vi "MAIN_HGB2_rev04.vi"() -> ()   [LabVIEW 2016]
uses:
  Producer_Case_Structure.ctl
  Consumer Control.ctl
  <vilib>/Utility/error.llb/DialogType.ctl
  <vilib>/DAQmx/write.llb/DAQmx Write (Analog 1D DBL NChan 1Samp).vi
  <vilib>/DAQmx/miscellaneous.llb/DAQmx Fill In Error Info.vi
  <vilib>/express/express analysis/Spectral/Block/exnSpectralBlock spectral measurements RMS poly.vi
  <vilib>/express/express analysis/Spectral/Block/exnSpectralBlock spectral measurements RMS array WFM.vi
  <vilib>/express/express analysis/Spectral/XNode/ExpressSpectralMeasurementsBlockNode.xnode
panel:
  in  "Dummy Variable 2":dbl=100.0
  in  "Evaluate\nShutdown\nCriteria":bool
  out "TDMS":i32=28826
  out "Acc":i32
  in  "Numeric":i32
  out "Producer":i32=163974
  out "Control":i32=5963
  in  "Speed Setpoint":dbl
  in  "Operator Notes":string
  in  "Dummy Variable":dbl
  in  "Record Data":bool
  in  "Sample Rate [S/s]":dbl=10.0
  in  "file path":path=path "C:/LabVIEW/TDMS Data/raw/090921-LifeTest1.tdms"
  in  "Stop":bool
  in  "Tab Control":T1(tab)=enum."Pressure & Temperature"
  out "System Temperatures":waveform(dbl)[](graph)=[{"t0"=timestamp(3713989500.4597507 s since 1904-01-01), "dt"=0.1, "Y"=[59.13780420730835, 59.13780420730835, 59.13780420730835, 59.13780420730835, 59.13780420730835], "attributes"=variant("NI_ChannelName"=variant(string "T_dis_dwnstrm"), "NI_UnitDescription"=variant(string "Deg C"))}, {"t0"=timestamp(3713989500.4597507 s since 1904-01-01), "dt"=0.1, "Y"=[19.89625827807839, 19.89625827807839, 19.89625827807839, 19.89625827807839, 19.89625827807839], "attributes"=variant("NI_ChannelName"=variant(string "T_liq"), "NI_UnitDescription"=variant(string "Deg C"))}, {"t0"=timestamp(3713989500.4597507 s since 1904-01-01), "dt"=0.1, "Y"=[51.99833247781037, 51.99833247781037, 51.99833247781037, 51.99833247781037, 51.99833247781037], "attributes"=variant("NI_ChannelName"=variant(string "T_gas_mix"), "NI_UnitDescription"=variant(string "Deg C"))}, {"t0"=timestamp(3713989500.4597507 s since 1904-01-01), "dt"=0.1, "Y"=[19.22760588195371, 19.22760588195371, 19.22760588195371, 19.22760588195371, 19.22760588195371], "attributes"=variant("NI_ChannelName"=variant(string "T_wf_cd_out"), "NI_UnitDescription"=variant(string "Deg C"))}, {"t0"=timestamp(3713989500.4597507 s since 1904-01-01), "dt"=0.1, "Y"=[18.627060719483154, 18.627060719483154, 18.627060719483154, 18.627060719483154, 18.627060719483154], "attributes"=variant("NI_ChannelName"=variant(string "T_cf_in"), "NI_UnitDescription"=variant(string "Deg C"))}]
  out "System Pressures":waveform(dbl)[](graph)=[{"t0"=timestamp(3713989500.4597507 s since 1904-01-01), "dt"=0.1, "Y"=[578.0486646128056, 578.0682722227018, 578.1264189279104, 578.222428603953, 578.1051210068165], "attributes"=variant("NI_ChannelName"=variant(string "P_comp_suc"))}, {"t0"=timestamp(3713989500.4597507 s since 1904-01-01), "dt"=0.1, "Y"=[583.306176195375, 583.3785215845983, 583.209828363933, 583.2270695548225, 583.3612803937087], "attributes"=variant("NI_ChannelName"=variant(string "P_comp_dis"))}, {"t0"=timestamp(3713989500.4597507 s since 1904-01-01), "dt"=0.1, "Y"=[578.9482116510878, 578.9603819034805, 578.9117008939097, 578.9999352237569, 578.9603819034805], "attributes"=variant("NI_ChannelName"=variant(string "P_comp_int"))}]
  out "Mass Flow":waveform(dbl)(graph)={"t0"=timestamp(3713989500.4597507 s since 1904-01-01), "dt"=0.1, "Y"=[-2.9024525025681674e-05, -2.9024525025681674e-05, -2.884801084886493e-05, -2.874504424572183e-05, -2.8818591819395473e-05], "attributes"=variant("NI_ChannelName"=variant(string "m_dot_wf"))}
  out "Setpoint Temperatures":waveform(dbl)[](graph)=[{"t0"=timestamp(3713989500.4597507 s since 1904-01-01), "dt"=0.1, "Y"=[31.196546478325374, 31.196546478325374, 31.196546478325374, 31.196546478325374, 31.196546478325374], "attributes"=variant("NI_ChannelName"=variant(string "T_comp_suc"), "NI_UnitDescription"=variant(string "Deg C"))}, {"t0"=timestamp(3713989500.4597507 s since 1904-01-01), "dt"=0.1, "Y"=[50.404968165402465, 50.404968165402465, 50.404968165402465, 50.404968165402465, 50.404968165402465], "attributes"=variant("NI_ChannelName"=variant(string "T_comp_out"), "NI_UnitDescription"=variant(string "Deg C"))}, {"t0"=timestamp(3713989500.4597507 s since 1904-01-01), "dt"=0.1, "Y"=[10.877218299088199, 10.876120226653185, 10.872864039787359, 10.867488088099194, 10.874056684092338], "attributes"=variant("NI_ChannelName"=variant(string "Suc_Suph"), "NI_UnitDescription"=variant(string "Deg C"))}]
  out "Power Constituents":waveform(dbl)[](graph)=[{"t0"=timestamp(3713989500.4597507 s since 1904-01-01), "dt"=0.1, "Y"=[-0.3841233029528297, -0.3841233029528297, -0.38402523952126444, -0.384466524963301, -0.3847116835422213], "attributes"=variant("NI_ChannelName"=variant(string "Voltage"))}, {"t0"=timestamp(3713989500.4597507 s since 1904-01-01), "dt"=0.1, "Y"=[-0.033083011419059005, -0.033507952955837084, -0.03358967248214029, -0.03337720171375125, -0.03327913828218598], "attributes"=variant("NI_ChannelName"=variant(string "Frequency"))}, {"t0"=timestamp(3713989499.86075 s since 1904-01-01), "dt"=0.1, "Y"=[0.07524272613227367, 0.09587410651147366, 0.12166333198547363, 0.09587410651147366, 0.07524272613227367], "attributes"=variant("NI_ChannelName"=variant(string "Torque"))}, {"t0"=timestamp(3713989499.910749 s since 1904-01-01), "dt"=0.1, "Y"=[-11.165670305490494, 3.2762959599494934, 13.591986149549484, 13.591986149549484, 1.2131579220294952], "attributes"=variant("NI_ChannelName"=variant(string "Tachometer"))}]
  out "Raw Acceleration":waveform(dbl)[](graph)
  out "Accel. Spectrum":cluster{"f0":dbl, "df":dbl, "magnitude":dbl[]}[](graph)
  in  "?":path=path "C:/Users/ASITest/Desktop/REFPROP"
  in  "Working Fluid":string="R134A.FLD"
  # "Stop VI"
  # "Air Squared Hot Gas Bypass Test Stand"
  # "Point to where REFPROP is..."
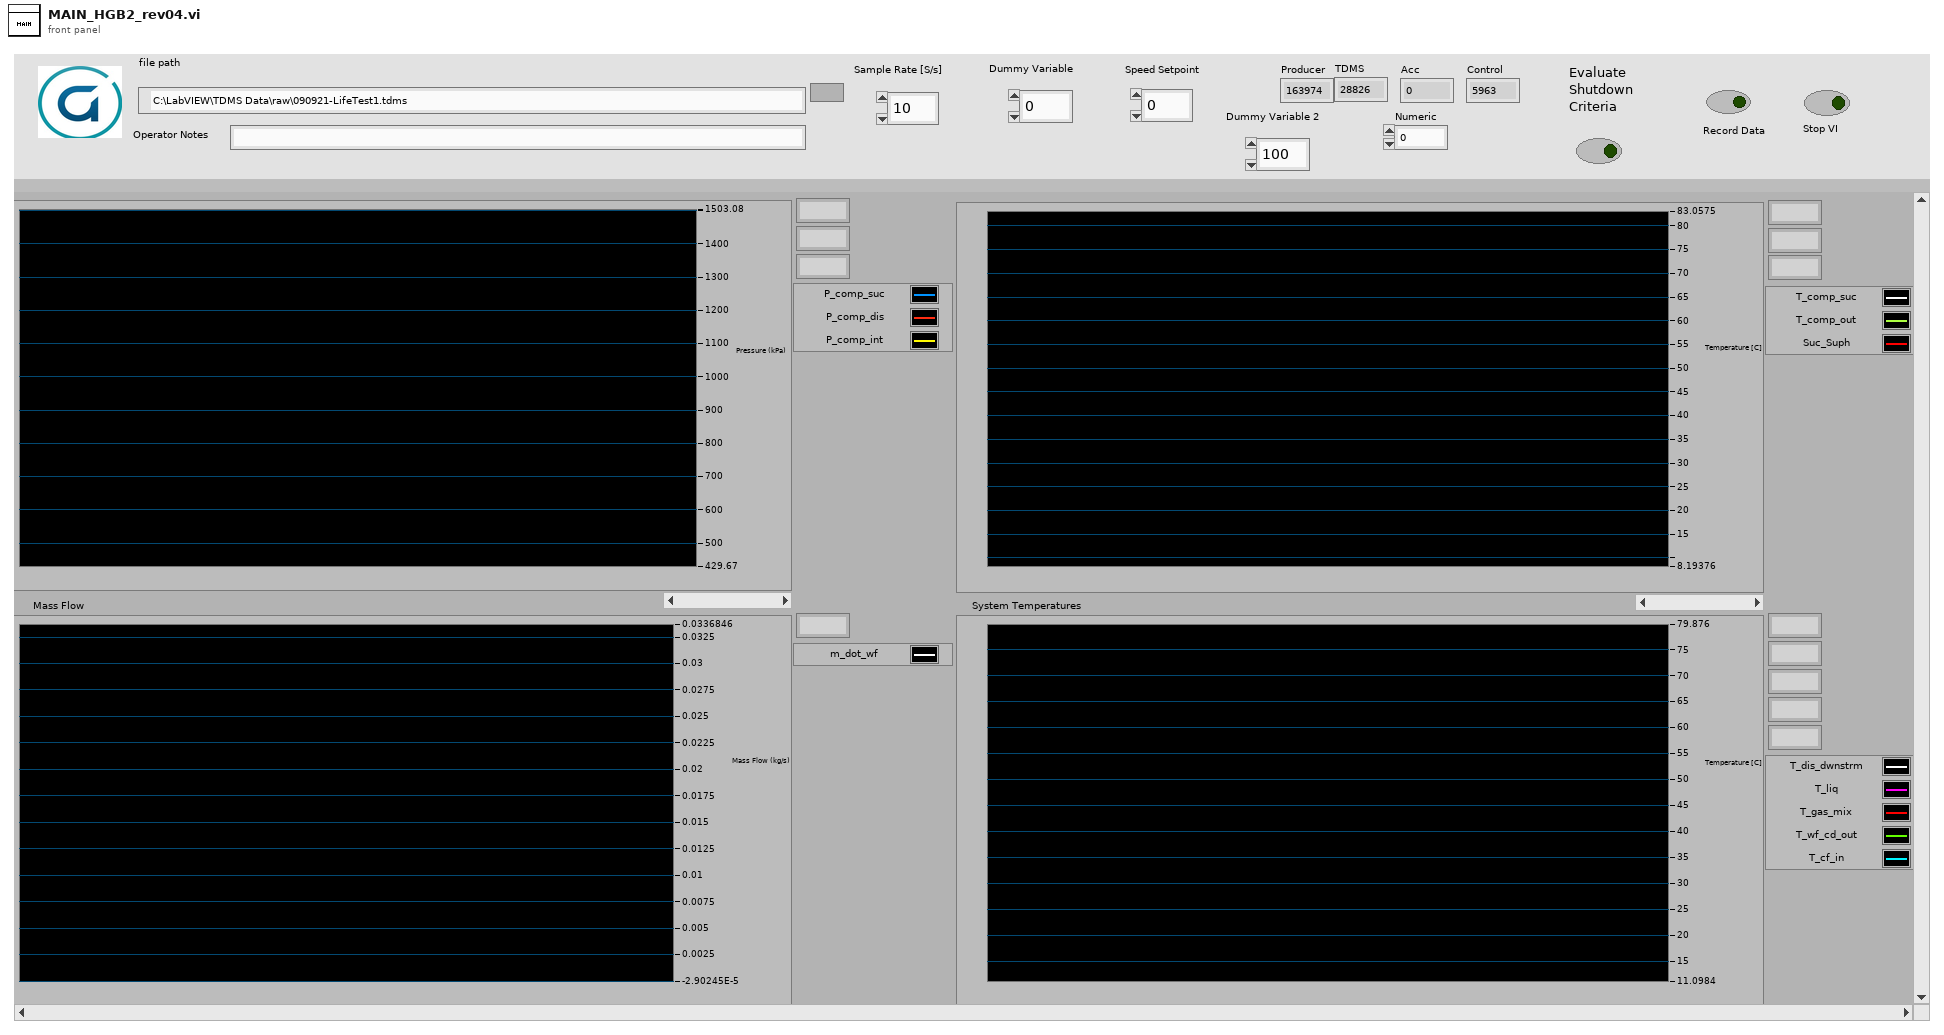
[diagram p1: front panel]
types:
  T1 = enum32{"Schematic", "Pressure & Temperature", "Power", "Acceleration", "Efficiency"}
  T2 = typedef "Consumer Control.ctl" = enum16{"System Run", "Shutdown"}
  T3 = enum16{"open", "open or create", "create or replace", "create", "open (read-only)"}
  T4 = typedef "Producer_Case_Structure.ctl" = enum16{"Initialize", "Read", "Write", "Display", "Queue", "Evaluate", "Error", "Shutdown"}
  T5 = cluster{"Data Main":waveform(dbl)[], "Accelerometer":waveform(dbl)[], "Dummy Variable":dbl, "Operator Notes":string, "Speed Setpoint":dbl, "NI 6001":waveform(dbl)[], "On/Off":dbl}
  T6 = typedef "DialogType.ctl" = u16
  T7 = cluster{"averaging mode":u16, "weighting mode":u16, "number of averages":u32}
  T8 = cluster{"dB On (F)":bool, "unwrap phase (F)":bool, "convert to degree (F)":bool}
  T9 = cluster{"All Channels":tag[], "All Labels":string[], "All Units":string[], "Slope":dbl[], "Y-Intercept":dbl[]}
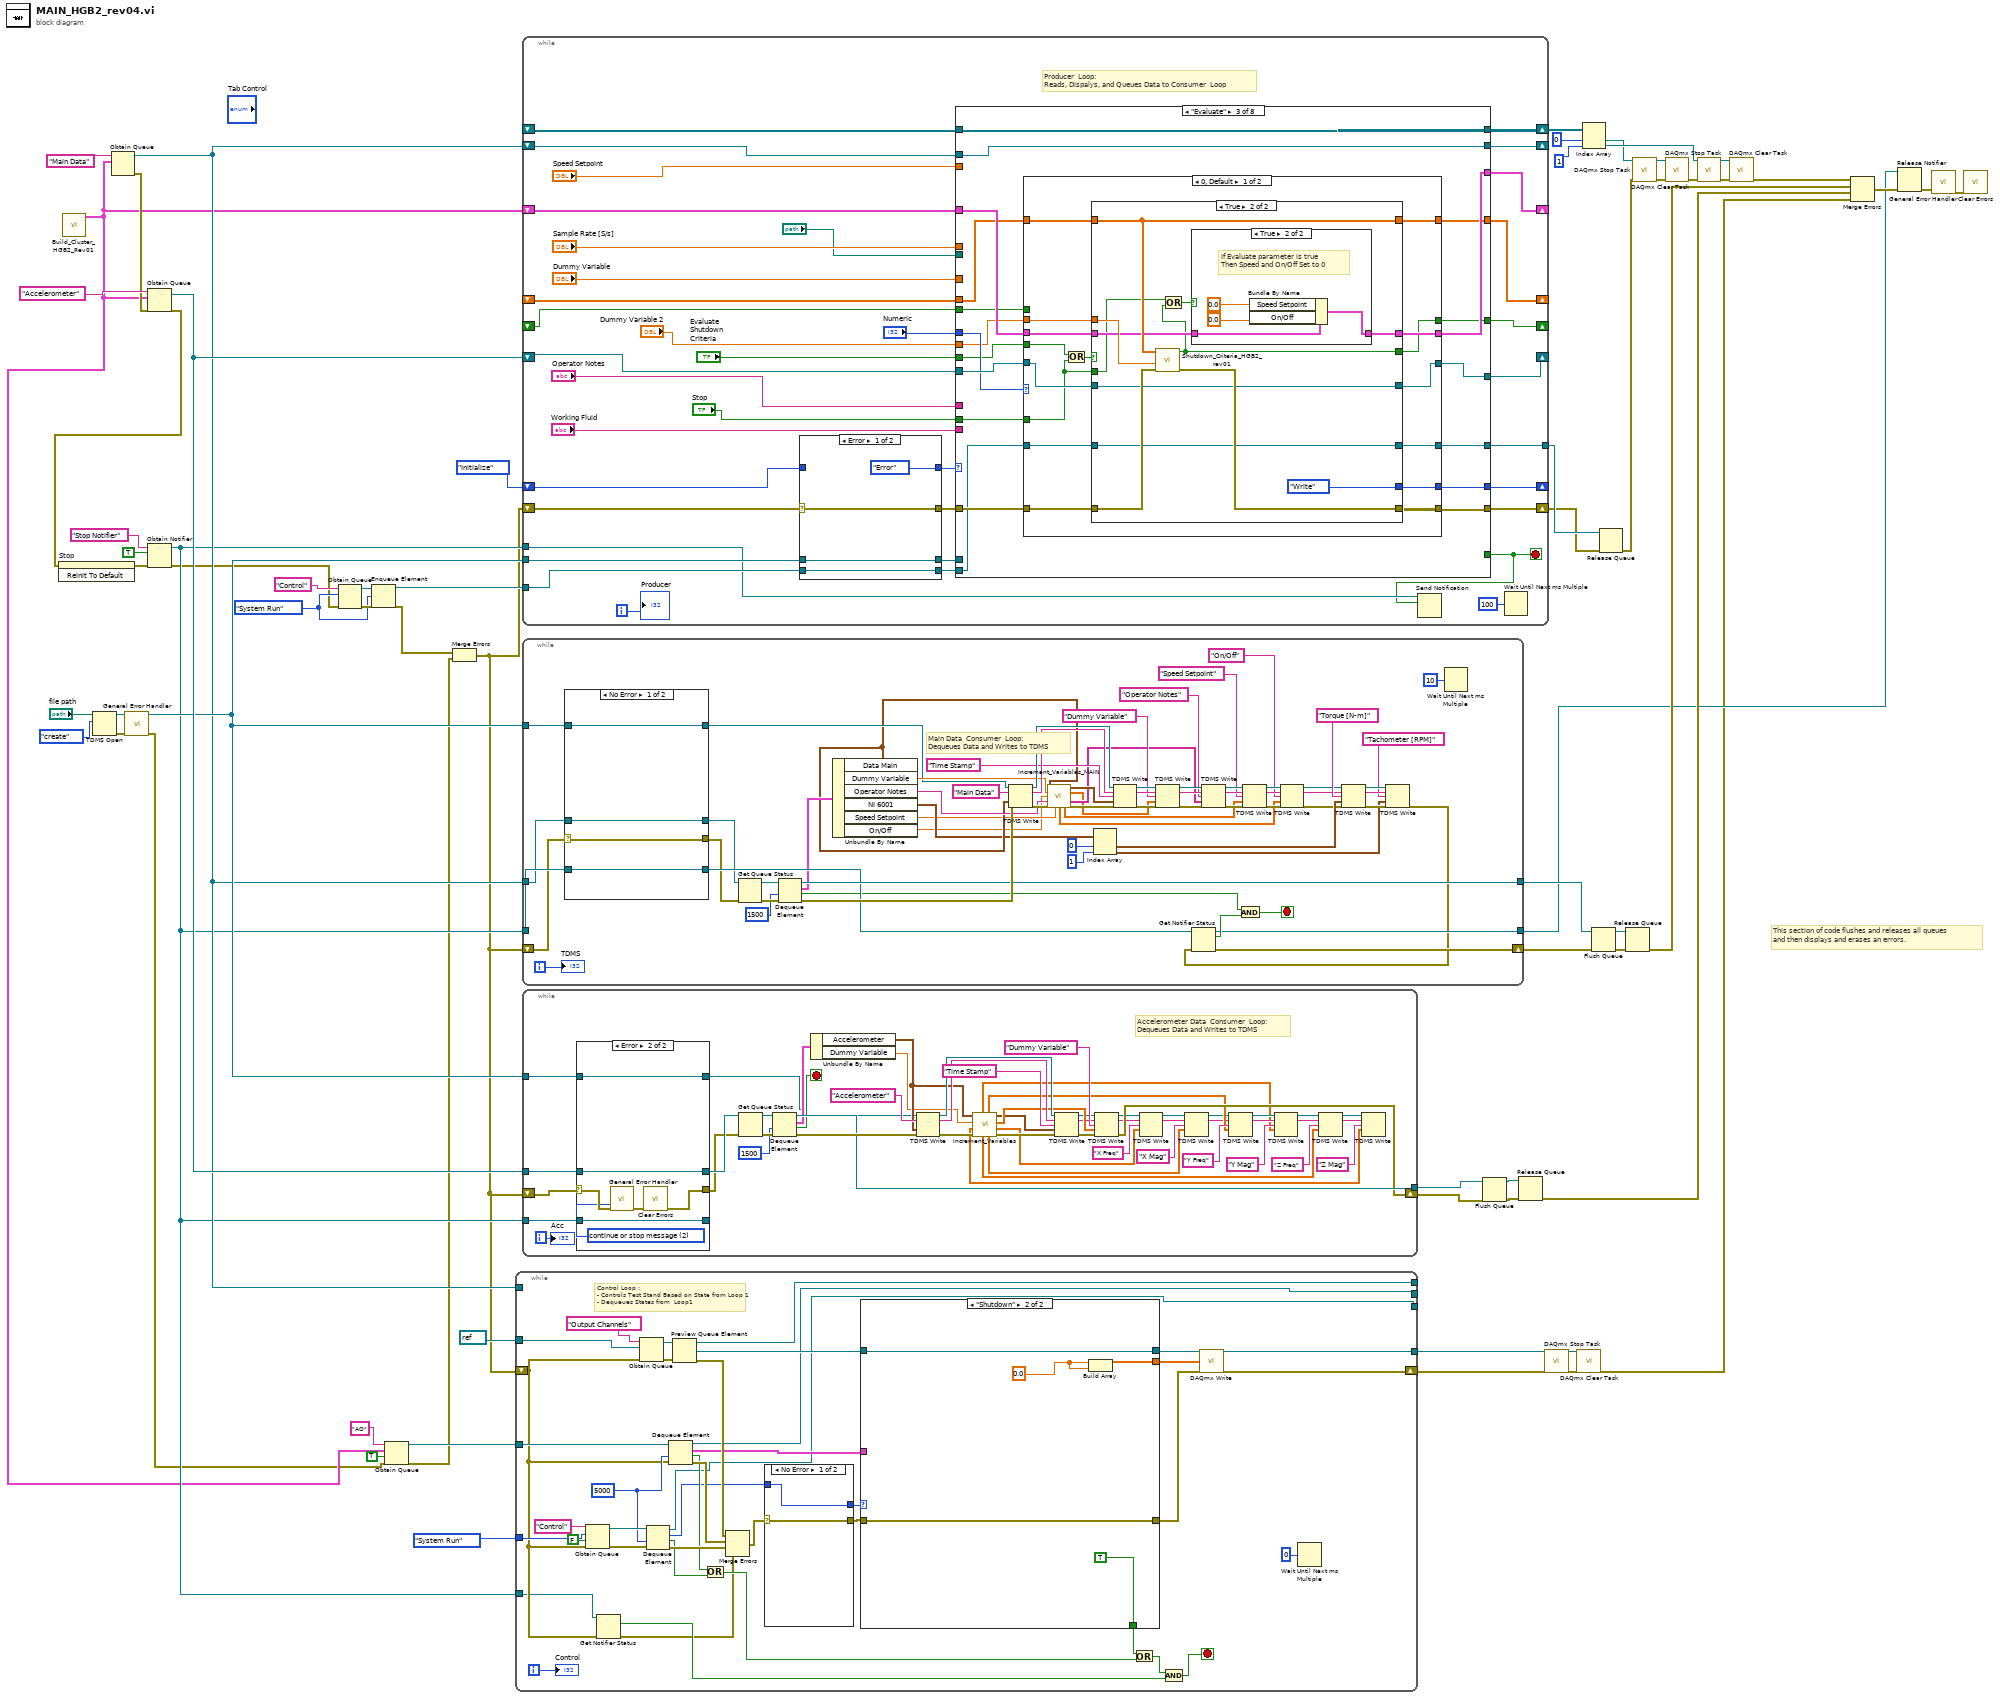
[diagram p0: block diagram]
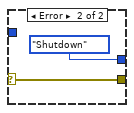
[diagram p2: hidden frame]
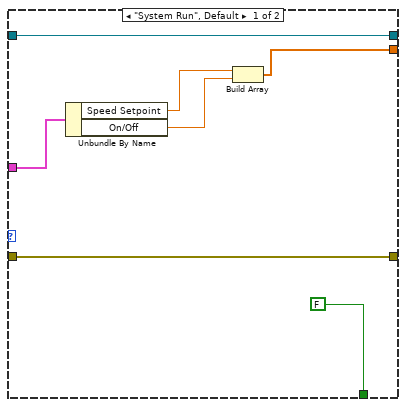
[diagram p3: hidden frame]
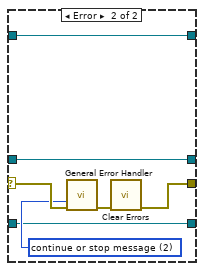
[diagram p5: hidden frame]
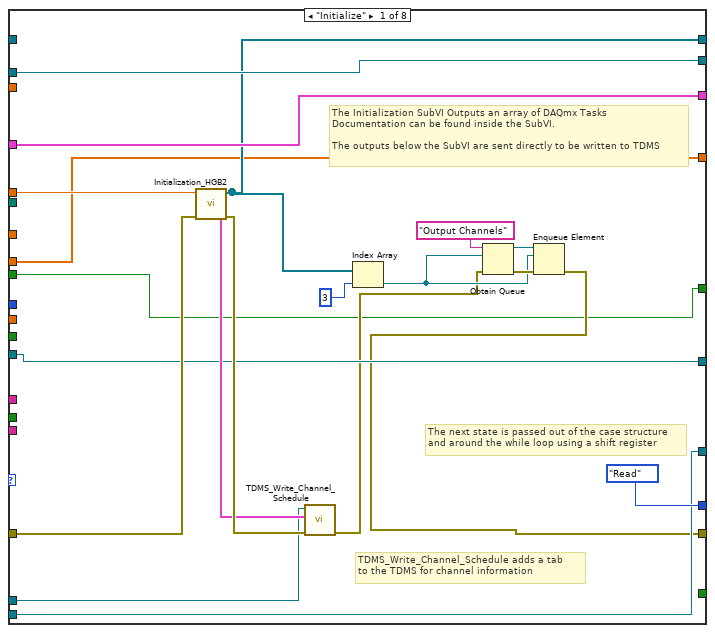
[diagram p6: hidden frame]
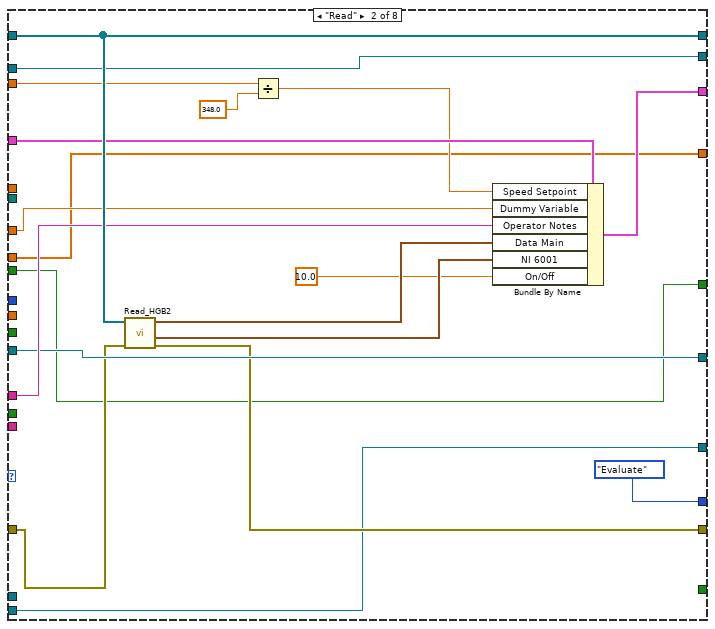
[diagram p7: hidden frame]
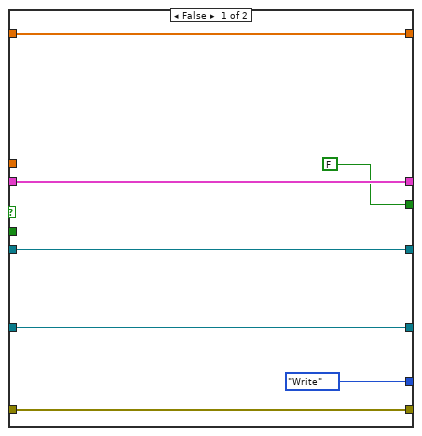
[diagram p8: hidden frame]
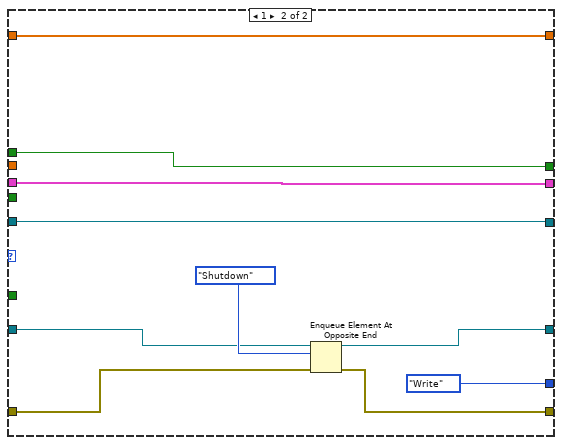
[diagram p10: hidden frame]
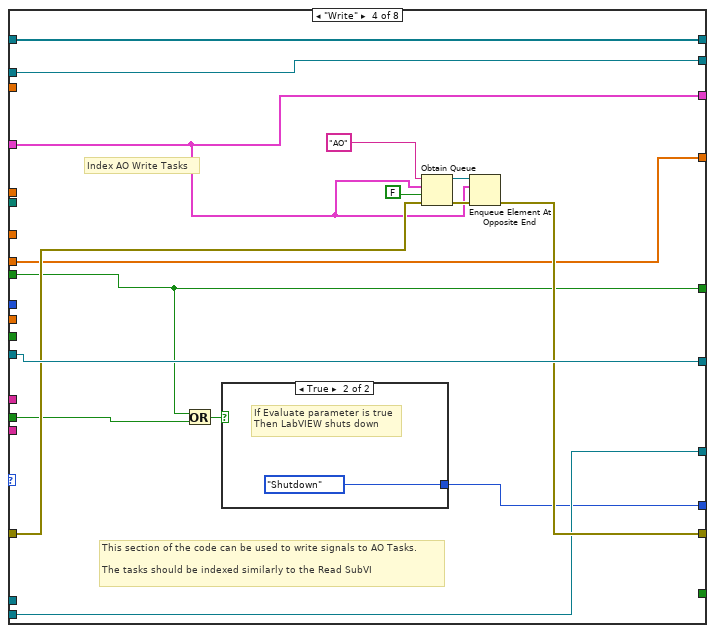
[diagram p11: hidden frame]
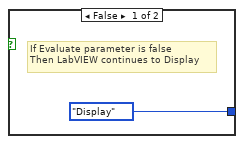
[diagram p12: hidden frame]
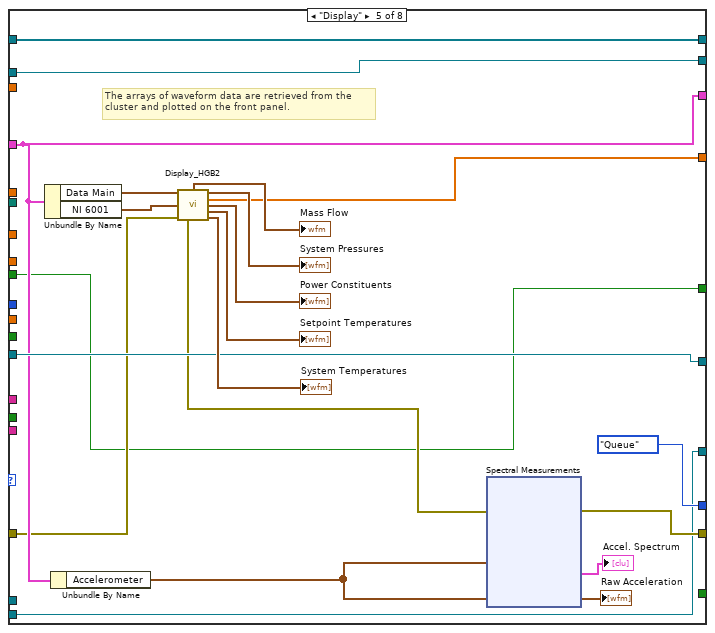
[diagram p13: hidden frame]
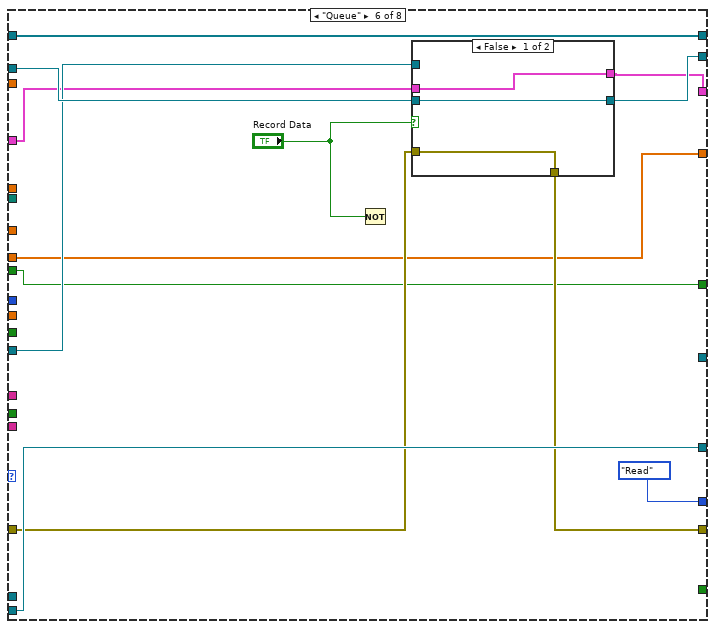
[diagram p14: hidden frame]
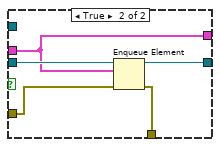
[diagram p15: hidden frame]
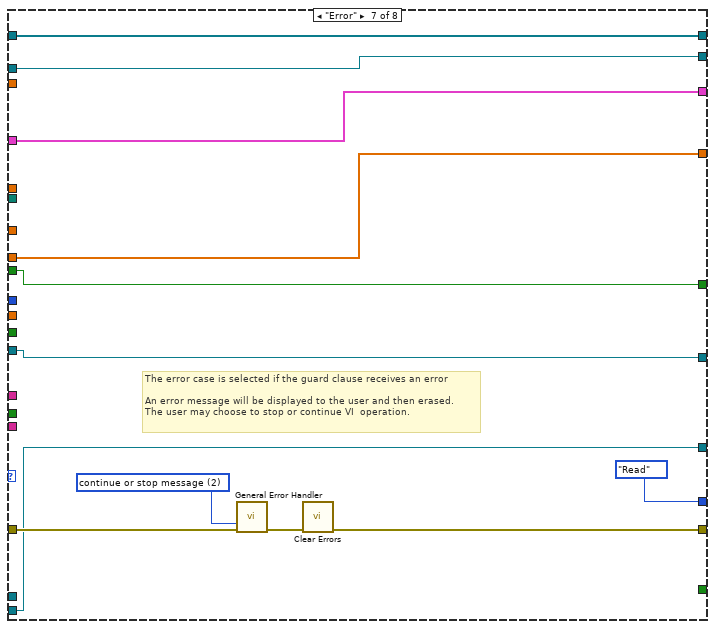
[diagram p16: hidden frame]
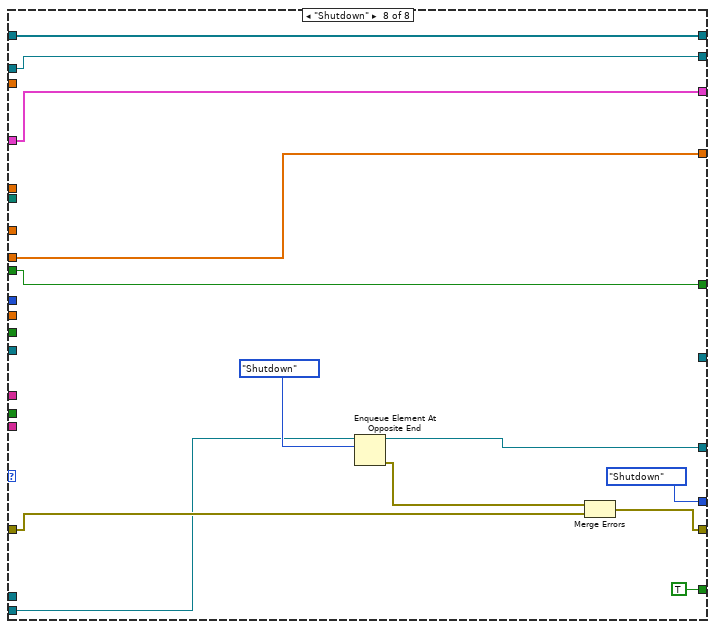
[diagram p17: hidden frame]
diagram:
  w21 = Consumer_Control."System Run"
  # "This section of code flushes and releases all queues \nand then displays and erases an errors."
  n1 = call "Build_Cluster_HGB2_Rev01.vi"() -> ("output cluster"=w13:T5)  [unwired: 11 in]
  n2 = TDMS Open(10:T3."create" ("operation (0:open)"), 11:"file path") -> (0:w54:errorcluster, 3:w37:refnum<k34>)  [unwired: 5 in]
  n3 = Obtain Queue(name (unnamed)="Main Data", element data type=w13) -> (queue out=w34:refnum<queue>, error out=w43:errorcluster)  [unwired: 3 in, 1 out]
  n4 = call <vilib>:"General Error Handler.vi"("error in (no error)"=w54) -> ("error out"=w12:errorcluster)  [unwired: 10 in, 4 out]
  n5 = Obtain Queue(name (unnamed)="Accelerometer", element data type=w13, error in (no error)=w43) -> (queue out=w42:refnum<queue>, error out=w11:errorcluster)  [unwired: 2 in, 1 out]
  n6 = invoke on="Stop" class="Bool (strict)" method="Reinit To Default"(error in=w11) -> (error out=w59:errorcluster)  [unwired: 2 in, 2 out]
  n7 = Obtain Notifier(name (unnamed)="Stop Notifier", notification data type=TRUE, error in (no error)=w59) -> (notifier out=w30:refnum<notifier>, error out=w10:errorcluster)  [unwired: 1 in, 1 out]
  n8 = Obtain Queue(name (unnamed)="Control", element data type=w21, error in (no error)=w10) -> (queue out=w23:refnum<queue>, error out=w22:errorcluster)  [unwired: 2 in, 1 out]
  n9 = Enqueue Element(queue=w23, element=w21, error in (no error)=w22) -> (queue out=w20:refnum<queue>, error out=w8:errorcluster)  [unwired: 1 in, 1 out]
  n10 = Obtain Queue(name (unnamed)="AO", element data type=w13, create if not found? (T)=TRUE, error in (no error)=w12) -> (queue out=w14:refnum<queue>, error out=w7:errorcluster)  [unwired: 1 in, 1 out]
  n11 = Merge Errors(w8, w7) -> (w9:errorcluster)
  n12 = while {
    tunnel: [w102] -> w4
    shift-right: [w89] -> w3
    shift-left: w9 -> [w70]
    tunnel: refnum<k21> refnum ("task in") -> [w97]
    tunnel: w34 -> [_]
    tunnel: Consumer_Control."System Run" -> [w87]
    tunnel: w30 -> [w69]
    tunnel: [w74] -> _
    tunnel: [w73] -> _
    tunnel: [w72] -> _
    tunnel: w14 -> [w71]
    i -> [w79]
    stop <- w68 stop-if-true
    w92 = 5000 ("timeout in ms (-1)")
    # "Control Loop :\n- Controls Test Stand Based on State from Loop 1\n- Dequeues States from  Loop1"
    n13 = Obtain Queue(name (unnamed)="Control", element data type=w87, create if not found? (T)=FALSE, error in (no error)=w70) -> (queue out=w101:refnum<queue>, error out=w93:errorcluster)  [unwired: 1 in, 1 out]
    n14 = Get Notifier Status(notifier=w69, error in (no error)=w70) -> (current notification=w66:bool, error out=w65:errorcluster)  [unwired: 3 out]
    n15 = Obtain Queue(name (unnamed)="Output Channels", element data type=w97, error in (no error)=w70) -> (queue out=w98:refnum<queue>, error out=w96:errorcluster)  [unwired: 2 in, 1 out]
    n16 = Dequeue Element(queue=w101, timeout in ms (-1)=w92, error in (no error)=w93) -> (queue out=w72:refnum<queue>, element=w86:T2, timed out?=w90:bool, error out=w94:errorcluster)
    n17 = Dequeue Element(queue=w71, timeout in ms (-1)=w92, error in (no error)=w70) -> (queue out=w73:refnum<queue>, element=w80:T5, timed out?=w91:bool, error out=w95:errorcluster)
    n18 = Preview Queue Element(queue=w98, error in (no error)=w96) -> (queue out=w74:refnum<queue>, element=w99:refnum<k21>, error out=w88:errorcluster)  [unwired: 1 in, 1 out]
    n19 = Or(x=w91, y=w90) -> (x .or. y?=w77:bool)
    n20 = Merge Errors(w88, w95, w94, w65) -> (w85:errorcluster)
    n21 = case shown="No Error" w85 {
      selector: w85 -> [w106 w108]
      tunnel: [w106 w108] -> w84
      tunnel: w86 -> [w105 _]
      tunnel: [w105 Consumer_Control."Shutdown"] -> w83
      frame No Error {
      }
      frame Error {
      }
    }
    n22 = case shown="\"Shutdown\"" w83 {
      tunnel: w99 -> [w115 w119]
      tunnel: [w110 w120] -> w104
      tunnel: [w115 w119] -> w103
      tunnel: w80 -> [w112 _]
      tunnel: w84 -> [w113 w117]
      tunnel: [FALSE TRUE] -> w78
      tunnel: [w113 w117] -> w82
      frame "System Run", Default {
        n23 = Unbundle By Name(w112) -> ("Speed Setpoint"=w111:dbl, "On/Off"=w109:dbl)
        n24 = Build Array(w111, w109) -> (w110:dbl[])
      }
      frame "Shutdown" {
        w116 = 0.0 ("Speed Setpoint 2")
        n25 = Build Array(w116, w116) -> (w120:dbl[])
      }
    }
    n26 = Or(x=w78, y=w77) -> (x .or. y?=w67:bool)
    n27 = And(x=w67, y=w66) -> (x .and. y?=w68:bool)
    n28 = call-poly <vilib>:"DAQmx Write.vi"("task/channels in"=w103, "data"=w104, "error in"=w82) -> ("task out"=w102:refnum<k21>, "error out"=w89:errorcluster)  [unwired: 10 in, 1 out]
    n29 = Wait Until Next ms Multiple(millisecond multiple=u32 0) -> ()  [unwired: 1 out]
    "Control" <- w79
  }
  n30 = while {
    tunnel: w37 -> [w175]
    tunnel: [w185] -> w51
    tunnel: w34 -> [w176]
    tunnel: w30 -> [w178]
    shift-right: [w183] -> w26
    shift-left: w9 -> [w174]
    tunnel: [w153] -> w25
    i -> [w138]
    stop <- w180 stop-if-true
    # "Main Data  Consumer  Loop: \nDequeues Data and Writes to TDMS"
    n31 = case shown="No Error" w174 {
      selector: w174 -> [w191 w197]
      tunnel: [w191 w196] -> w156
      tunnel: w178 -> [w190 w192]
      tunnel: [w190 w192] -> w179
      tunnel: [w189 w194] -> w177
      tunnel: w176 -> [w189 w194]
      tunnel: [w188 w193] -> w154
      tunnel: w175 -> [w188 w193]
      frame No Error {
      }
      frame Error {
        w195 = T6 2 items=["no dialog", "OK message", "continue or stop message", "OK message + warnings", "continue/stop + warnings"] ("type of dialog (OK msg:1)")
        n32 = call <vilib>:"General Error Handler.vi"("type of dialog (OK msg:1)"=w195, "error in (no error)"=w197) -> ("error out"=w198:errorcluster)  [unwired: 9 in, 4 out]
        n33 = call <vilib>:"Clear Errors.vi"("error in (no error)"=w198) -> ("error out"=w196:errorcluster)  [unwired: 5 in, 1 out]
      }
    }
    n34 = Get Queue Status(queue=w177, error in (no error)=w156) -> (queue out=w182:refnum<queue>, error out=w186:errorcluster)  [unwired: 1 in, 6 out]
    n35 = Dequeue Element(queue=w182, timeout in ms (-1)=1500, error in (no error)=w186) -> (queue out=w185:refnum<queue>, element=w155:T5, timed out?=w173:bool, error out=w187:errorcluster)
    n36 = Unbundle By Name(w155) -> ("Data Main"=w145:waveform(dbl)[], "Dummy Variable"=w163:dbl, "Operator Notes"=w151:string, "NI 6001"=w140:waveform(dbl)[], "Speed Setpoint"=w139:dbl, "On/Off"=w123:dbl)
    n37 = TDMS Write(0:w154, 5:"Main Data" ("group name in (Untitled)"), 9:w145, 11:w187) -> (4:w170:refnum<k34>, 6:w168:string, 15:w171:errorcluster)  [unwired: 2 in, 1 out]
    n38 = call "Increment_Variables_MAIN.vi"("Data Main"=w145, "Dummy Variable"=w163, "On/Off"=w123, "Operator Notes"=w151, "error in 2"=w171, "Speed Setpoint"=w139) -> ("Time Stamp"=w164:timestamp[], "Dummy Variable Array"=w141:dbl[], "Operator Notes Array"=w152:string[], "On/Off Array"=w122:dbl[], "Speed Setpoint Array"=w147:dbl[], "error IO"=w172:errorcluster)  [unwired: 4 in]
    n39 = Index Array(array=w140, index #1=0 ("index"), index #2=1 ("index")) -> (element #1=w142:waveform(dbl), element #2=w130:waveform(dbl))
    n40 = TDMS Write(0:w170, 5:w168, 7:"Time Stamp" ("group name in (Untitled)"), 9:w164, 11:w172) -> (4:w167:refnum<k34>, 6:w165:string, 15:w166:errorcluster)  [unwired: 1 in, 1 out]
    n41 = TDMS Write(0:w167, 5:w165, 7:"Dummy Variable" ("group name in (Untitled)"), 9:w141, 11:w166) -> (4:w161:refnum<k34>, 6:w160:string, 15:w162:errorcluster)  [unwired: 1 in, 1 out]
    n42 = TDMS Write(0:w161, 5:w160, 7:"Operator Notes" ("group name in (Untitled)"), 9:w152, 11:w162) -> (4:w148:refnum<k34>, 6:w149:string, 15:w150:errorcluster)  [unwired: 1 in, 1 out]
    n43 = TDMS Write(0:w148, 5:w149, 7:"Speed Setpoint" ("group name in (Untitled)"), 9:w147, 11:w150) -> (4:w129:refnum<k34>, 6:w128:string, 15:w127:errorcluster)  [unwired: 1 in, 1 out]
    n44 = TDMS Write(0:w129, 5:w128, 7:"On/Off" ("channel name(s) in (Untitled)"), 9:w122, 11:w127) -> (4:w125:refnum<k34>, 6:w124:string, 15:w126:errorcluster)  [unwired: 1 in, 1 out]
    n45 = TDMS Write(0:w125, 5:w124, 7:"Torque [N-m]" ("channel name(s) in (Untitled)"), 9:w142, 11:w126) -> (4:w132:refnum<k34>, 6:w133:string, 15:w135:errorcluster)  [unwired: 1 in, 1 out]
    n46 = TDMS Write(0:w132, 5:w133, 7:"Tachometer [RPM]" ("channel name(s) in (Untitled)"), 9:w130, 11:w135) -> (15:w134:errorcluster)  [unwired: 1 in, 3 out]
    n47 = Get Notifier Status(notifier=w179, error in (no error)=w134) -> (notifier out=w153:refnum<notifier>, current notification=w184:bool, error out=w183:errorcluster)  [unwired: 2 out]
    n48 = And(x=w173, y=w184) -> (x .and. y?=w180:bool)
    n49 = Wait Until Next ms Multiple(millisecond multiple=u32 10) -> ()  [unwired: 1 out]
    "TDMS" <- w138
  }
  n50 = while {
    shift-right: [w231] -> _
    shift-left: Producer_Case_Structure."Initialize" ("Enum") -> [w200]
    shift-right: [w233] -> w56
    shift-left: _ -> [w232]
    tunnel: w30 -> [w210]
    shift-right: [w230] -> _
    shift-left: w13 -> [w229]
    shift-right: [w228] -> _
    shift-left: w34 -> [w227]
    shift-right: [w234] -> w18
    shift-left: w9 -> [w209]
    tunnel: w37 -> [w222]
    shift-right: [w220] -> _
    shift-left: w42 -> [w221]
    tunnel: w20 -> [w215]
    tunnel: [w213] -> w19
    shift-right: [w207] -> _
    shift-left: _ -> [w206]
    shift-right: [w203] -> _
    shift-left: _ -> [w202]
    i -> [w216]
    stop <- w204 stop-if-true
    # "Producer  Loop: \nReads, Dispalys, and Queues Data to Consumer  Loop"
    n51 = case shown="Error" w209 {
      selector: w209 -> [w441 w445]
      tunnel: [w441 w445] -> w235
      tunnel: [w440 w444] -> w223
      tunnel: w222 -> [w440 w444]
      tunnel: w215 -> [w439 w443]
      tunnel: [w439 w443] -> w214
      tunnel: w200 -> [_ w442]
      tunnel: [Producer_Case_Structure."Error" ("Enum") w442] -> w199
      frame Error {
      }
      frame No Error {
      }
    }
    n52 = case shown="\"Evaluate\"" w199 {
      tunnel: w235 -> [w255 w262 w291 w354 w366 w395 w421 w435]
      tunnel: [w238 w265 w290 w356 w374 w394 w418 w434] -> w234
      tunnel: [w243 w273 w286 w359 w380 w403 w422 w431] -> w233
      tunnel: w232 -> [_ w273 w286 w359 w380 w403 w422 w431]
      tunnel: [Producer_Case_Structure."Read" ("Enum") Producer_Case_Structure."Evaluate" ("Enum") w282 w347 Producer_Case_Structure."Queue" ("Enum") Producer_Case_Structure."Read" ("Enum") Producer_Case_Structure."Read" ("Enum") Producer_Case_Structure."Shutdown" ("Enum")] -> w231
      tunnel: [_ _ _ _ _ _ _ TRUE ("Stop")] -> w204
      tunnel: [w251 w271 w292 w349 w373 w400 w420 w429] -> w230
      tunnel: w229 -> [w251 w267 w293 w349 w373 w398 w420 w429]
      tunnel: [w253 w272 w287 w358 w378 w401 w417 w430] -> w228
      tunnel: w227 -> [w253 w272 w287 w358 w378 w402 w417 w430]
      tunnel: "Sample Rate [S/s]" -> [w252 _ _ _ _ _ _ _]
      tunnel: "Dummy Variable" -> [_ w268 _ _ _ _ _ _]
      tunnel: "Operator Notes" -> [_ w270 _ _ _ _ _ _]
      tunnel: w223 -> [w248 _ _ _ _ _ _ _]
      tunnel: w221 -> [w247 w269 w285 w357 w376 w399 w416 _]
      tunnel: [w247 w269 w284 w357 w376 _ w416 _] -> w220
      tunnel: "?" -> [_ _ _ _ _ _ _ _]
      tunnel: "Working Fluid" -> [_ _ _ _ _ _ _ _]
      tunnel: "Speed Setpoint" -> [_ w260 _ _ _ _ _ _]
      tunnel: w214 -> [w240 w263 w289 w355 w365 w396 w415 w433]
      tunnel: [w240 w263 w288 w355 w365 w396 w415 w432] -> w213
      tunnel: "Numeric" -> [_ _ w283 _ _ _ _ _]
      tunnel: "Evaluate\nShutdown\nCriteria" -> [_ _ w278 _ _ _ _ _]
      tunnel: [w237 w258 w280 w348 w364 w393 w414 w426] -> w207
      tunnel: w206 -> [w237 w258 w281 w348 _ w393 w414 w426]
      tunnel: "Dummy Variable 2" -> [_ _ w279 _ _ _ _ _]
      tunnel: [w236 w257 w277 w345 w362 w392 w413 w425] -> w203
      tunnel: w202 -> [w236 w257 w276 w345 w362 w392 w413 w425]
      tunnel: "Stop" -> [_ _ w275 w344 _ _ _ _]
      frame "Initialize" {
        # "TDMS_Write_Channel_Schedule adds a tab \nto the TDMS for channel information"
        # "The next state is passed out of the case structure \nand around the while loop using a shift register"
        # "The Initialization SubVI Outputs an array of DAQmx Tasks\nDocumentation can be found inside the SubVI.\n\nThe outputs below the SubVI are sent directly to be written to TDMS"
        n53 = call "Initialization_HGB2.vi"("error in"=w255, "Sample Rate"=w252) -> ("error out"=w250:errorcluster, "Task Array"=w243:refnum<k21>[], "output cluster"=w249:T9)  [unwired: 7 in]
        n54 = call "TDMS_Write_Channel_Schedule.vi"("error in (no error)"=w250, "output cluster"=w249, "Refnum in"=w248) -> ("error out"=w239:errorcluster)  [unwired: 8 in]
        n55 = Index Array(array=w243, index=3) -> (element=w241:refnum<k21>)
        n56 = Obtain Queue(name (unnamed)="Output Channels", element data type=w241, error in (no error)=w239) -> (queue out=w245:refnum<queue>, error out=w244:errorcluster)  [unwired: 2 in, 1 out]
        n57 = Enqueue Element(queue=w245, element=w241, error in (no error)=w244) -> (error out=w238:errorcluster)  [unwired: 1 in, 2 out]
      }
      frame "Read" {
        n58 = call "Read_HGB2.vi"("error in (no error)"=w262, "Task Array"=w273) -> ("error out"=w265:errorcluster, "NI 6001"=w264:waveform(dbl)[], "Data Main"=w266:waveform(dbl)[])  [unwired: 7 in]
        n59 = Divide(x=w260, y=348.0) -> (x/y=w259:dbl)
        n60 = Bundle By Name(cluster=w267, "Speed Setpoint"=w259, "Dummy Variable"=w268, "Operator Notes"=w270, "Data Main"=w266, "NI 6001"=w264, "On/Off"=10.0) -> (w271:T5)
      }
      frame "Evaluate" {
        n61 = case shown="0, Default" w283 {
          tunnel: w293 -> [w305 w343]
          tunnel: [w304 w343] -> w292
          tunnel: w291 -> [w309 w339]
          tunnel: [w307 w338] -> w290
          tunnel: w289 -> [w299 w341]
          tunnel: [w298 w340] -> w288
          tunnel: [w303 w337] -> w284
          tunnel: w285 -> [w302 w337]
          tunnel: [w306 Producer_Case_Structure."Write" ("Enum")] -> w282
          tunnel: w281 -> [w300 w335]
          tunnel: [w301 w335] -> w280
          tunnel: w279 -> [w308 _]
          tunnel: w278 -> [w295 _]
          tunnel: [w297 w334] -> w277
          tunnel: w276 -> [_ w334]
          tunnel: w275 -> [w294 _]
          frame 0, Default {
            n62 = Or(x=w295, y=w294) -> (x .or. y?=w296:bool)
            n63 = case shown="True" w296 {
              tunnel: w300 -> [w316 w324]
              tunnel: w309 -> [w313 w328]
              tunnel: w308 -> [_ w327]
              tunnel: [w313 w326] -> w307
              tunnel: [Producer_Case_Structure."Write" ("Enum") Producer_Case_Structure."Write" ("Enum")] -> w306
              tunnel: w305 -> [w315 w320]
              tunnel: [w315 w321] -> w304
              tunnel: [w314 w325] -> w303
              tunnel: w302 -> [w314 w325]
              tunnel: [w316 w324] -> w301
              tunnel: w299 -> [w312 w323]
              tunnel: [w312 w323] -> w298
              tunnel: [FALSE ("Boolean") w318] -> w297
              tunnel: w294 -> [_ w317]
              frame False {
              }
              frame True {
                n64 = call "Shutdown_Criteria_HGB2_rev01.vi"("error in (no error)"=w328, "Dummy Variable 2"=w327, "Data Array"=w324) -> ("error out"=w326:errorcluster, "Boolean"=w318:bool)  [unwired: 7 in]
                n65 = Or(x=w317, y=w318) -> (x .or. y?=w319:bool)
                n66 = case shown="True" w319 {
                  tunnel: [w329 w330] -> w321
                  tunnel: w320 -> [w329 w331]
                  frame False {
                    # "If Evaluate parameter is false\nThen cluster is NOT altered"
                  }
                  frame True {
                    # "If Evaluate parameter is true\nThen Speed and On/Off Set to 0"
                    n67 = Bundle By Name(cluster=w331, "Speed Setpoint"=0.0, "On/Off"=0.0) -> (w330:T5)
                  }
                }
              }
            }
          }
          frame 1 {
            n68 = Enqueue Element At Opposite End(queue=w341, element=Consumer_Control."Shutdown", error in (no error)=w339) -> (queue out=w340:refnum<queue>, error out=w338:errorcluster)  [unwired: 1 in, 1 out]
          }
        }
      }
      frame "Write" {
        # "This section of the code can be used to write signals to AO Tasks.\n\nThe tasks should be indexed similarly to the Read SubVI"
        # "Index AO Write Tasks"
        n69 = Or(x=w345, y=w344) -> (x .or. y?=w346:bool)
        n70 = case shown="True" w346 {
          tunnel: [Producer_Case_Structure."Display" ("Enum") Producer_Case_Structure."Shutdown" ("Enum")] -> w347
          frame False {
            # "If Evaluate parameter is false\nThen LabVIEW continues to Display"
          }
          frame True {
            # "If Evaluate parameter is true\nThen LabVIEW shuts down"
          }
        }
        n71 = Obtain Queue(name (unnamed)="AO", element data type=w349, create if not found? (T)=FALSE, error in (no error)=w354) -> (queue out=w352:refnum<queue>, error out=w353:errorcluster)  [unwired: 1 in, 1 out]
        n72 = Enqueue Element At Opposite End(queue=w352, element=w349, error in (no error)=w353) -> (error out=w356:errorcluster)  [unwired: 1 in, 2 out]
      }
      frame "Display" {
        # "The arrays of waveform data are retrieved from the \ncluster and plotted on the front panel."
        n73 = Unbundle By Name(w373) -> ("Data Main"=w371:waveform(dbl)[], "NI 6001"=w367:waveform(dbl)[])
        n74 = Unbundle By Name(w373) -> ("Accelerometer"=w372:waveform(dbl)[])
        "Raw Acceleration" <- w372
        n75 = call "Display_HGB2.vi"("data"=w371, "NI 6001"=w367, "error in (no error)"=w366) -> ("Mass Flow"=→"Mass Flow":waveform(dbl), "System Pressures"=→"System Pressures":waveform(dbl)[], "Data Array"=w364:dbl[], "Power Constituents"=→"Power Constituents":waveform(dbl)[], "Setpoint Temperatures"=→"Setpoint Temperatures":waveform(dbl)[], "error out"=w375:errorcluster, "System Temperatures"=→"System Temperatures":waveform(dbl)[])  [unwired: 6 in]
        n76 = xnode "Spectral Measurements"("Signals"=w372, "error in (no error)"=w375) -> ("FFT - (RMS)"=→"Accel. Spectrum":cluster{"f0":dbl, "df":dbl, "magnitude":dbl[]}[], "error out"=w374:errorcluster)  [unwired: 1 out]
      }
      frame "Queue" {
        n77 = Not(x="Record Data") -> ()  [unwired: 1 out]
        n78 = case shown="False" "Record Data" {
          tunnel: w398 -> [w406 w410]
          tunnel: w402 -> [w407 w411]
          tunnel: [w407 w412] -> w401
          tunnel: [w406 w410] -> w400
          tunnel: w399 -> [_ _]
          tunnel: w395 -> [w405 w409]
          tunnel: [w405 w408] -> w394
          frame False {
          }
          frame True {
            n79 = Enqueue Element(queue=w411, element=w410, error in (no error)=w409) -> (queue out=w412:refnum<queue>, error out=w408:errorcluster)  [unwired: 1 in, 1 out]
          }
        }
      }
      frame "Error" {
        w423 = T6 2 items=["no dialog", "OK message", "continue or stop message", "OK message + warnings", "continue/stop + warnings"] ("type of dialog (OK msg:1)")
        # "The error case is selected if the guard clause receives an error\n\nAn error message will be displayed to the user and then erased. \nThe user may choose to stop or continue VI  operation."
        n80 = call <vilib>:"General Error Handler.vi"("type of dialog (OK msg:1)"=w423, "error in (no error)"=w421) -> ("error out"=w419:errorcluster)  [unwired: 9 in, 4 out]
        n81 = call <vilib>:"Clear Errors.vi"("error in (no error)"=w419) -> ("error out"=w418:errorcluster)  [unwired: 5 in, 1 out]
      }
      frame "Shutdown" {
        n82 = Enqueue Element At Opposite End(queue=w433, element=Consumer_Control."Shutdown") -> (queue out=w432:refnum<queue>, error out=w436:errorcluster)  [unwired: 2 in, 1 out]
        n83 = Merge Errors(w436, w435) -> (w434:errorcluster)
      }
    }
    n84 = Send Notification(notification=w204, notifier=w210) -> ()  [unwired: 1 in, 2 out]
    n85 = Wait Until Next ms Multiple(millisecond multiple=u32 100) -> ()  [unwired: 1 out]
    "Producer" <- w216
  }
  n86 = while {
    tunnel: w37 -> [w491]
    tunnel: [w497] -> w39
    tunnel: w42 -> [w492]
    tunnel: w30 -> [w494]
    shift-right: [w472] -> w36
    shift-left: w9 -> [w490]
    i -> [w446]
    stop <- w471 stop-if-true
    # "Accelerometer Data  Consumer  Loop: \nDequeues Data and Writes to TDMS"
    n87 = case shown="Error" w490 {
      selector: w490 -> [w503 w509]
      tunnel: [w503 w508] -> w482
      tunnel: w494 -> [w502 w504]
      tunnel: [w502 w504] -> _
      tunnel: [w501 w506] -> w493
      tunnel: w492 -> [w501 w506]
      tunnel: [w500 w505] -> w480
      tunnel: w491 -> [w500 w505]
      frame No Error {
      }
      frame Error {
        w507 = T6 2 items=["no dialog", "OK message", "continue or stop message", "OK message + warnings", "continue/stop + warnings"] ("type of dialog (OK msg:1)")
        n88 = call <vilib>:"General Error Handler.vi"("type of dialog (OK msg:1)"=w507, "error in (no error)"=w509) -> ("error out"=w510:errorcluster)  [unwired: 9 in, 4 out]
        n89 = call <vilib>:"Clear Errors.vi"("error in (no error)"=w510) -> ("error out"=w508:errorcluster)  [unwired: 5 in, 1 out]
      }
    }
    n90 = Get Queue Status(queue=w493, error in (no error)=w482) -> (queue out=w496:refnum<queue>, error out=w498:errorcluster)  [unwired: 1 in, 6 out]
    n91 = Dequeue Element(queue=w496, timeout in ms (-1)=1500, error in (no error)=w498) -> (queue out=w497:refnum<queue>, element=w481:T5, timed out?=w471:bool, error out=w499:errorcluster)
    n92 = Unbundle By Name(w481) -> ("Accelerometer"=w484:waveform(dbl)[], "Dummy Variable"=w479:dbl)
    n93 = TDMS Write(0:w480, 5:"Accelerometer" ("group name in (Untitled)"), 9:w484, 11:w499) -> (4:w487:refnum<k34>, 6:w485:string, 15:w488:errorcluster)  [unwired: 2 in, 1 out]
    n94 = call "Increment_Variables.vi"("error in 2"=w488, "Dummy Variable"=w479, "Accelerometer"=w484) -> ("error IO"=w489:errorcluster, "X Accel Freq Array"=w468:dbl[], "Dummy Variable Array"=w477:dbl[], "Time Stamp"=w473:timestamp[], "X Accel Mag Array"=w466:dbl[], "Y Accel Freq Array"=w449:dbl[], "Z Accel Freq Array"=w451:dbl[], "Y Accel Mag Array"=w450:dbl[], "Z Accel Mag Array"=w452:dbl[])
    n95 = TDMS Write(0:w487, 5:w485, 7:"Time Stamp" ("group name in (Untitled)"), 9:w473, 11:w489) -> (4:w474:refnum<k34>, 6:w475:string, 15:w478:errorcluster)  [unwired: 1 in, 1 out]
    n96 = TDMS Write(0:w474, 5:w475, 7:"Dummy Variable" ("group name in (Untitled)"), 9:w477, 11:w478) -> (4:w469:refnum<k34>, 6:w470:string, 15:w472:errorcluster)  [unwired: 1 in, 1 out]
    n97 = TDMS Write(0:w469, 5:w470, 7:"X Freq" ("group name in (Untitled)"), 9:w468) -> (4:w463:refnum<k34>, 6:w464:string)  [unwired: 2 in, 2 out]
    n98 = TDMS Write(0:w463, 5:w464, 7:"X Mag" ("group name in (Untitled)"), 9:w466) -> (4:w448:refnum<k34>, 6:w447:string)  [unwired: 2 in, 2 out]
    n99 = TDMS Write(0:w448, 5:w447, 7:"Y Freq" ("group name in (Untitled)"), 9:w449) -> (4:w460:refnum<k34>, 6:w459:string)  [unwired: 2 in, 2 out]
    n100 = TDMS Write(0:w460, 5:w459, 7:"Y Mag" ("group name in (Untitled)"), 9:w450) -> (4:w461:refnum<k34>, 6:w462:string)  [unwired: 2 in, 2 out]
    n101 = TDMS Write(0:w461, 5:w462, 7:"Z Freq" ("group name in (Untitled)"), 9:w451) -> (4:w458:refnum<k34>, 6:w457:string)  [unwired: 2 in, 2 out]
    n102 = TDMS Write(0:w458, 5:w457, 7:"Z Mag" ("group name in (Untitled)"), 9:w452) -> ()  [unwired: 2 in, 4 out]
    "Acc" <- w446
  }
  n103 = Flush Queue(queue=w39, error in (no error)=w36) -> (queue out=w41:refnum<queue>, error out=w40:errorcluster)  [unwired: 1 out]
  n104 = Release Queue(queue=w41, error in (no error)=w40) -> (error out=w31:errorcluster)  [unwired: 1 in, 2 out]
  n105 = call <vilib>:"DAQmx Stop Task.vi"("task/channels in"=w4, "error in"=w3) -> ("task out"=w5:refnum<k21>, "error out"=w1:errorcluster)  [unwired: 12 in]
  n106 = call <vilib>:"DAQmx Clear Task.vi"("task in"=w5, "error in"=w1) -> ("error out"=w2:errorcluster)  [unwired: 13 in]
  n107 = Index Array(array=w56, index #1=0 ("index"), index #2=1 ("index")) -> (element #1=w35:refnum<k21>, element #2=w47:refnum<k21>)
  n108 = Flush Queue(queue=w51, error in (no error)=w26) -> (queue out=w52:refnum<queue>, error out=w50:errorcluster)  [unwired: 1 out]
  n109 = Release Queue(queue=w19, error in (no error)=w18) -> (error out=w17:errorcluster)  [unwired: 1 in, 2 out]
  n110 = Release Queue(queue=w52, error in (no error)=w50) -> (error out=w32:errorcluster)  [unwired: 1 in, 2 out]
  n111 = call <vilib>:"DAQmx Stop Task.vi"("task/channels in"=w35, "error in"=w17) -> ("task out"=w57:refnum<k21>, "error out"=w58:errorcluster)  [unwired: 12 in]
  n112 = call <vilib>:"DAQmx Clear Task.vi"("task in"=w57, "error in"=w58) -> ("error out"=w48:errorcluster)  [unwired: 13 in]
  n113 = call <vilib>:"DAQmx Stop Task.vi"("task/channels in"=w47, "error in"=w48) -> ("task out"=w45:refnum<k21>, "error out"=w49:errorcluster)  [unwired: 12 in]
  n114 = call <vilib>:"DAQmx Clear Task.vi"("task in"=w45, "error in"=w49) -> ("error out"=w6:errorcluster)  [unwired: 13 in]
  n115 = Merge Errors(w6, w32, w31, w2) -> (w28:errorcluster)
  n116 = Release Notifier(notifier=w25, error in (no error)=w28) -> (error out=w27:errorcluster)  [unwired: 1 in, 2 out]
  n117 = call <vilib>:"General Error Handler.vi"("error in (no error)"=w27) -> ("error out"=w38:errorcluster)  [unwired: 10 in, 4 out]
  n118 = call <vilib>:"Clear Errors.vi"("error in (no error)"=w38) -> ()  [unwired: 5 in, 2 out]
